vi "Matrix_SetRow.vi"(9 "Fill Row Vector":T1, 10 "Row":i32, 11 "input matrix":T1) -> (0 "Error":bool, 3 "output matrix":T1)   [LabVIEW 2019, in "Trajectory_Library.lvlib"]
doc: "Sets a row to a given row vector.\n \n\nInputs:\n - input matrix -- The input matrix\n - row -- The row to set.\n - val -- The row vector to set the given row to.\n\nOutputs:\n - output matrix -- resulting matrix\n - error -- If TRUE, an error occured."
uses:
  Trajectory_Library.lvlib
  <vilib>/Analysis/Matrix/Datatypes/RealMatrix.ctl
  MatBuilder_Create.vi
  <vilib>/Analysis/Matrix/NI_Matrix.lvlib
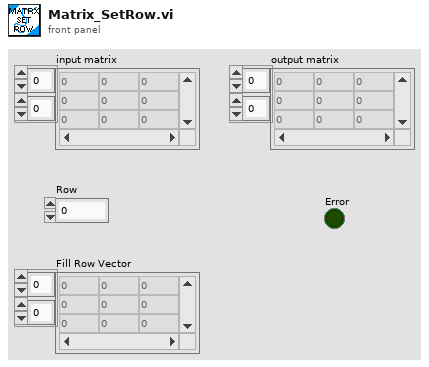
[diagram p1: front panel]
types:
  T1 = typedef "NI_Matrix.lvlib/RealMatrix.ctl" = dbl[][]
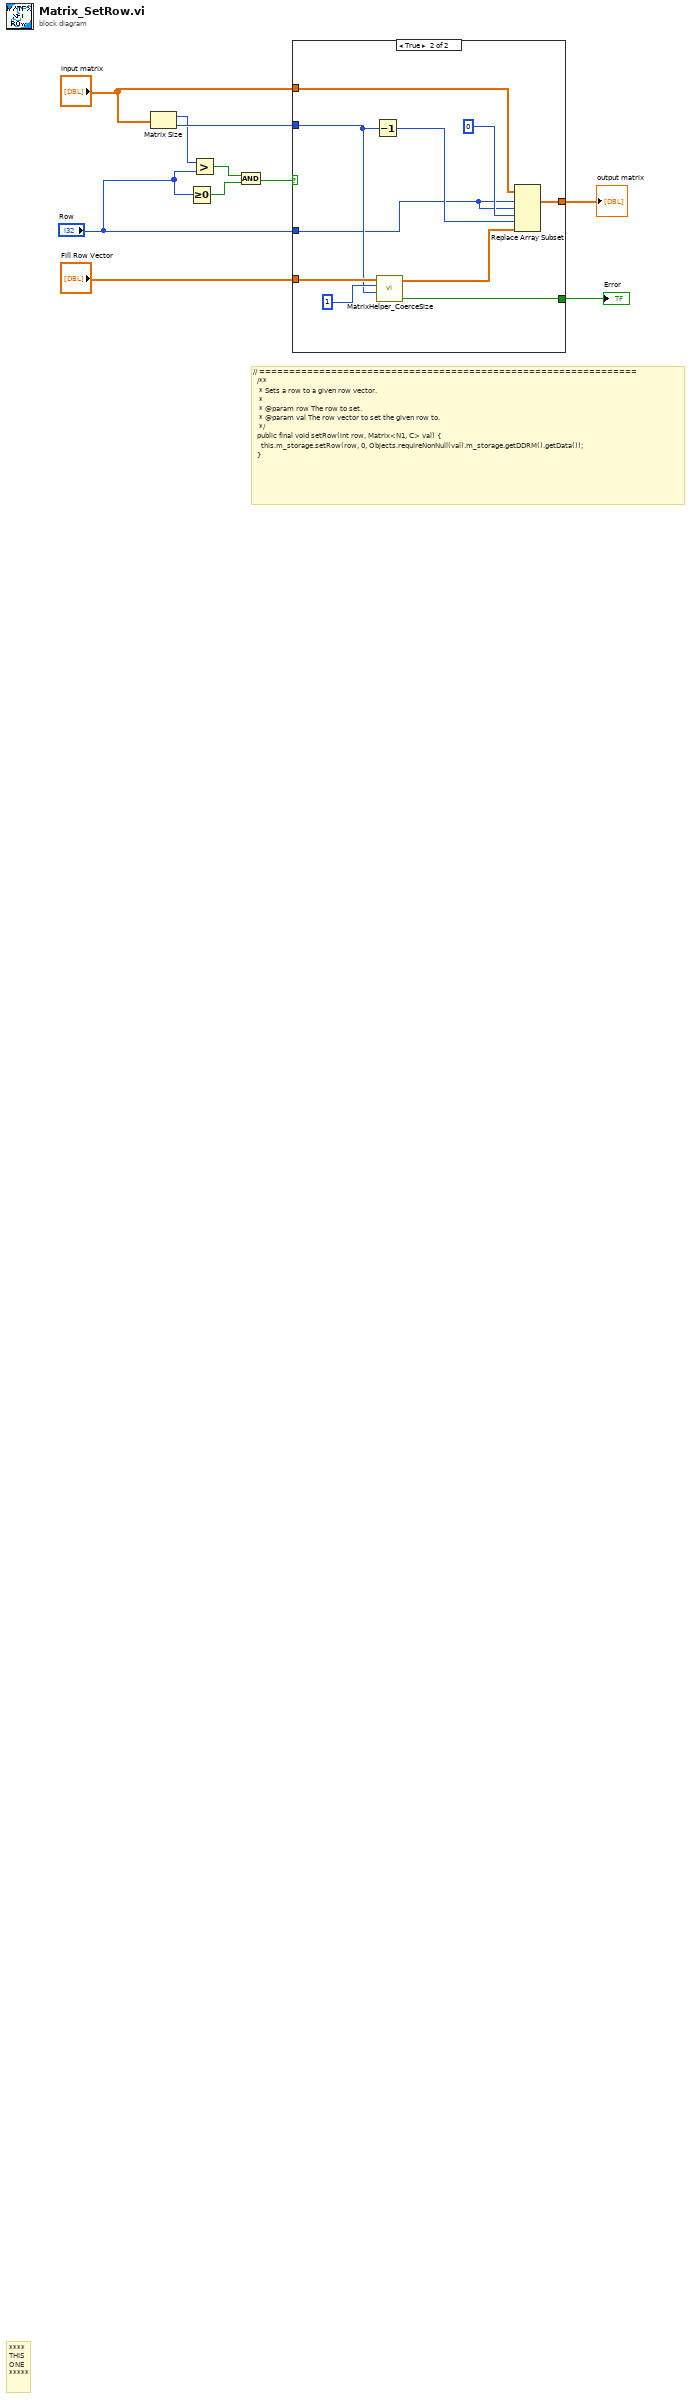
[diagram p0: block diagram]
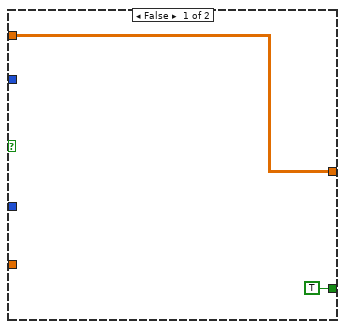
[diagram p2: hidden frame]
diagram:
  # "// ===============================================================\n  /**\n   * Sets a row to a given row vector.\n   *\n   * @param row The row to set.\n   * @param val The row vector to set the given row to.\n   */\n  public final void setRow(int row, Matrix<N1, C> val) {\n    this.m_storage.setRow(row, 0, Objects.requireNonNull(val).m_storage.getDDRM().getData());\n  }"
  # "****\nTHIS\nONE\n*****"
  n1 = Matrix Size(0:"input matrix") -> (1:w4:i32, 2:w7:i32)
  n2 = Greater Or Equal To 0?(x="Row") -> (x >= 0?=w5:bool)
  n3 = Greater?(x=w4, y="Row") -> (0:w6:bool)
  n4 = And(x=w6, y=w5) -> (x .and. y?=w1:bool)
  n5 = case shown="True" w1 {
    tunnel: "Fill Row Vector" -> [_ w22]
    tunnel: "input matrix" -> [w11 w21]
    tunnel: [w11 w19] -> w8
    tunnel: w7 -> [_ w17]
    tunnel: "Row" -> [_ w14]
    tunnel: [TRUE ("Coerced") w13] -> w2
    frame False {
    }
    frame True {
      n6 = Decrement(x=w17) -> (x-1=w15:i32)
      n7 = call "MatrixHelper_CoerceSize.vi"("Columns"=w17, "Rows"=1 ("Columns"), "input matrix"=w22) -> ("Coerced"=w13:bool, "output matrix"=w20:T1)  [unwired: 7 in]
      n8 = Replace Array Subset(array=w21, new element=w20, index (dim 0)=w14, index (dim 1)=w14, index (dim 2)=0 ("row 1"), index (dim 3)=w15) -> (w19:T1)
    }
  }
  "output matrix" <- w8
  "Error" <- w2
